vi "Generate Sine Wave.vi"() -> ()   [LabVIEW 2009]
uses:
  Controls/methodCall.ctl
  Controls/methodResponse.ctl
  XML-RPC Message Builder/Array/DoubleAsArray.vi
  XML-RPC Parser/GetScalarValue/ValueAsDouble.vi
  XML-RPC Parser/GetScalarValue/ValueAsInt.vi
  <vilib>/Analysis/NI_AALBase.lvlib
panel:
  in  "methodResponse":T1
  in  "timeout in ms":i32=100
  out "error out":errorcluster
  in  "methodCall":T2
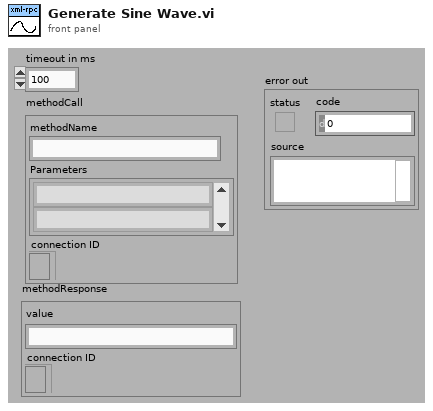
[diagram p1: front panel]
types:
  T1 = typedef "methodResponse.ctl" = cluster{"value":string, "connection ID":refnum<k5>}
  T2 = typedef "methodCall.ctl" = cluster{"methodName":string, "Parameters":string[], "connection ID":refnum<k5>}
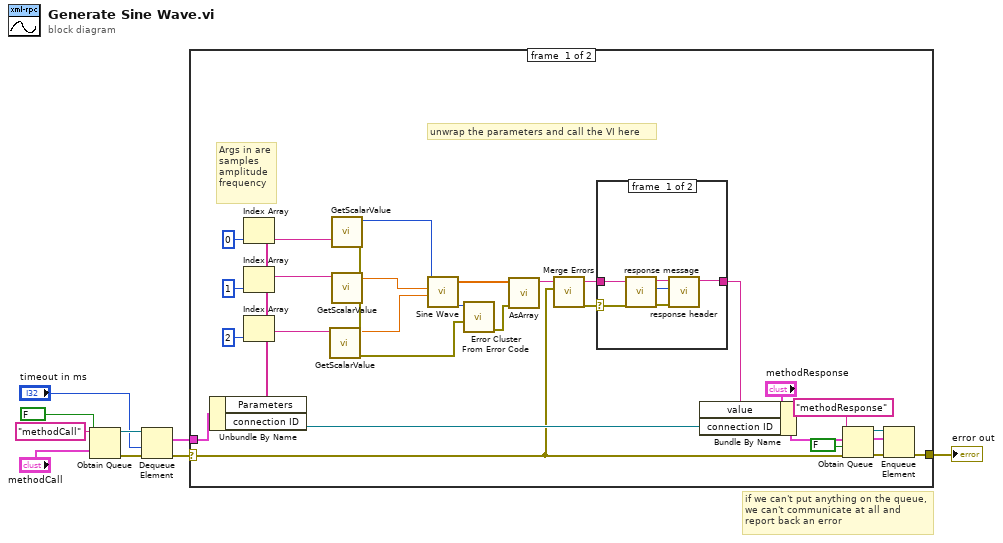
[diagram p0: block diagram]
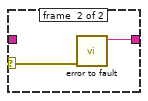
[diagram p2: hidden frame]
diagram:
  # "if we can't put anything on the queue, we can't communicate at all and report back an error"
  n1 = Obtain Queue(name (unnamed)="methodCall", element data type="methodCall", create if not found? (T)=FALSE) -> (queue out=w9:refnum<queue>, error out=w8:errorcluster)  [unwired: 2 in, 1 out]
  n2 = Dequeue Element(queue=w9, timeout in ms (-1)="timeout in ms", error in (no error)=w8) -> (element=w3:T2, error out=w4:errorcluster)  [unwired: 2 out]
  n3 = case shown="No Error" w4 {
    selector: w4 -> [w11 w48]
    tunnel: w3 -> [w39 _]
    tunnel: [w34 w48] -> w2
    frame #0 {
      # "Args in are\nsamples\namplitude\nfrequency"
      # "unwrap the parameters and call the VI here"
      n4 = Unbundle By Name(w39) -> ("Parameters"=w30:string[], "connection ID"=w31:refnum<k5>)
      n5 = Index Array(array=w30, index=0) -> (element=w26:string)
      n6 = Index Array(array=w30, index=1) -> (element=w23:string)
      n7 = Index Array(array=w30, index=2) -> (element=w20:string)
      n8 = call-poly "GetScalarValue.vi"("Parameter"=w26) -> ("error out"=w24:errorcluster, "value"=w25:i32)  [unwired: 9 in]
      n9 = call-poly "GetScalarValue.vi"("error in (no error)"=w24, "Parameter"=w23) -> ("error out"=w21:errorcluster, "value"=w22:dbl)  [unwired: 8 in]
      n10 = call-poly "GetScalarValue.vi"("error in (no error)"=w21, "Parameter"=w20) -> ("error out"=w16:errorcluster, "value"=w19:dbl)  [unwired: 8 in]
      n11 = call <vilib>:"Sine Wave.vi"("samples"=w25, "amplitude"=w22, "frequency"=w19) -> ("sine wave"=w18:dbl[], "error"=w17:i32)  [unwired: 2 in, 1 out]
      n12 = call <vilib>:"Error Cluster From Error Code.vi"("error in (no error)"=w16, "error code (0)"=w17) -> ("error out"=w15:errorcluster)  [unwired: 7 in]
      n13 = call-poly "AsArray.vi"("error in"=w15, "Array In"=w18) -> ("error out"=w13:errorcluster, "ArrayAsValue"=w14:string)  [unwired: 8 in]
      n14 = call <vilib>:"Merge Errors.vi"("error in 2 (no error)"=w11, "error in 1 (no error)"=w13) -> ("error out"=w12:errorcluster)  [unwired: 5 in]
      n15 = case shown="No Error" w12 {
        selector: w12 -> [w41 w47]
        tunnel: [w42 w46] -> w10
        tunnel: w14 -> [w45 _]
        frame #0 {
          n16 = call "response message.vi"("error in"=w41, "params (formatted)"=w45) -> ("error out"=w40:errorcluster, "length"=w43:i32, "response"=w44:string)  [unwired: 7 in]
          n17 = call "response header.vi"("error in"=w40, "Content-Length"=w43, "Content String"=w44) -> ("response string"=w42:string)  [unwired: 7 in, 1 out]
        }
        frame #1 {
          n18 = call "error to fault.vi"("error cluster"=w47) -> ("response string"=w46:string)  [unwired: 10 in]
        }
      }
      n19 = Bundle By Name(cluster="methodResponse", "value"=w10, "connection ID"=w31) -> (w32:T1)
      n20 = Obtain Queue(name (unnamed)="methodResponse", element data type=w32, create if not found? (T)=FALSE, error in (no error)=w11) -> (queue out=w35:refnum<queue>, error out=w36:errorcluster)  [unwired: 1 in, 1 out]
      n21 = Enqueue Element(queue=w35, element=w32, error in (no error)=w36) -> (error out=w34:errorcluster)  [unwired: 1 in, 2 out]
    }
    frame #1 {
    }
  }
  "error out" <- w2
